vi "Handle TCP Message.vi"(7 "TCPMessageAPI":refnum<class "TCPMessageAPI.lvclass">, 8 "error in (no error)":errorcluster, 10 "TcpPayload":T1, 11 "Vecto Message Bridge in":refnum<class "Vecto Message Bridge.lvclass">) -> (0 "error out":errorcluster, 3 "Vecto Message Bridge out":refnum<class "Vecto Message Bridge.lvclass">)   [LabVIEW 2020, in "Volatus.lvlib" / "Vecto Message Bridge.lvclass"]
uses:
  Vecto Message Bridge.lvclass
  lv-vecto/Vecto/TCPMessageService/TCPMessageAPI.lvclass
  messages/TcpPayload/Data.ctl
  Vecto Message Bridge.lvclass/Vecto Message Bridge.ctl
  MessageQ/MessageQ.lvclass/MessageQ.ctl
  MessageQ/MessageQ.lvclass
  messages/TcpPayload/TcpPayload.lvlib
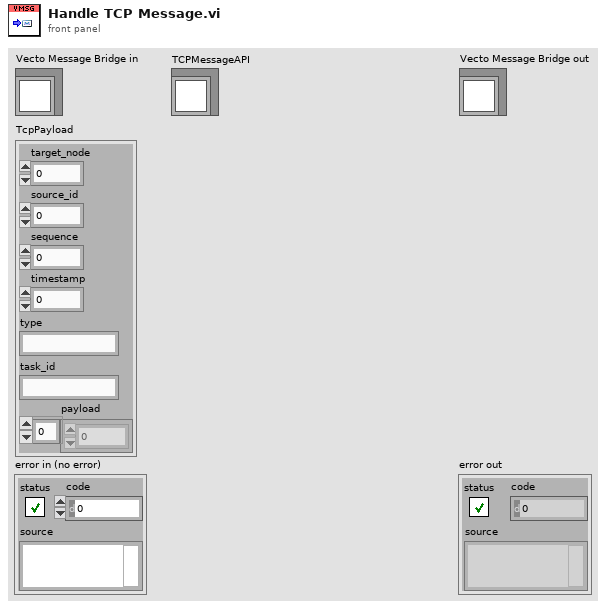
[diagram p1: front panel]
types:
  T1 = typedef "TcpPayload.lvlib/Data.ctl" = cluster{"target_node":u32, "source_id":u32, "sequence":u32, "timestamp":i64, "type":string, "task_id":string, "payload":u8[]}
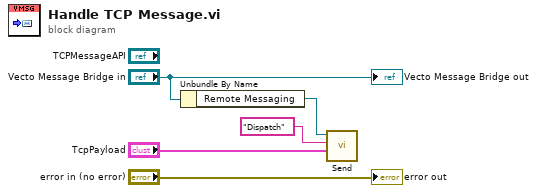
[diagram p0: block diagram]
diagram:
  n1 = Unbundle By Name("Vecto Message Bridge in") -> ("Remote Messaging"=w3:refnum<class "MessageQ.lvclass">)
  n2 = call "Send.vi"("Data"="TcpPayload", "ID"="Dispatch", "MessageQ in"=w3) -> ()  [unwired: 7 in, 2 out]
  "error out" <- "error in (no error)"
  "Vecto Message Bridge out" <- "Vecto Message Bridge in"
